vi "Apply Bounds.vi"(8 "error in":errorcluster, 10 "Bounds":refnum<class "Vec3d.lvclass">, 11 "Vec3d in":refnum<class "Vec3d.lvclass">) -> (0 "error out":errorcluster, 3 "Vec3d out":refnum<class "Vec3d.lvclass">)   [LabVIEW 2017, in "Vec3d.lvclass"]
doc: "Shrinks the vector if necessary so the magnitude of all components are less than the corresponding components of the Bounds Vec3d. All components are scaled equally so the direction of the vector will not change"
uses:
  Vec3d.lvclass
  Vec3d.lvclass/Vec3d.ctl
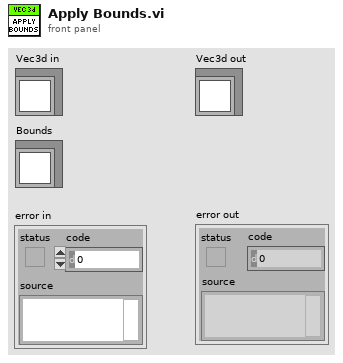
[diagram p1: front panel]
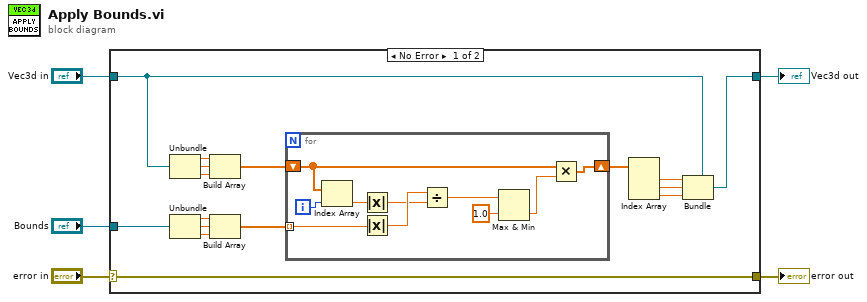
[diagram p0: block diagram]
diagram:
  n1 = case shown="No Error" "error in" {
    selector: "error in" -> [w21 w33]
    tunnel: [w21 w33] -> w4
    tunnel: [w6 w32] -> w2
    tunnel: "Vec3d in" -> [w7 w32]
    tunnel: "Bounds" -> [w20 _]
    frame No Error {
      n2 = Unbundle(w7) -> (w12:dbl, w14:dbl, w15:dbl)
      n3 = Unbundle(w20) -> (w19:dbl, w18:dbl, w17:dbl)
      n4 = Build Array(w12, w14, w15) -> (w13:dbl[])
      n5 = Build Array(w19, w18, w17) -> (w16:dbl[])
      n6 = for {
        tunnel: w16 -> [w30] mode=indexing
        shift-right: [w22] -> w11
        shift-left: w13 -> [w24]
        i -> [w31]
        n7 = Index Array(array=w24, index=w31) -> (element=w29:dbl)
        n8 = Absolute Value(x=w29) -> (abs(x)=w27:dbl)
        n9 = Absolute Value(x=w30) -> (abs(x)=w28:dbl)
        n10 = Divide(x=w28, y=w27) -> (x/y=w26:dbl)
        n11 = Max & Min(x=w26, y=1.0) -> (min(x,y)=w23:dbl)  [unwired: 1 out]
        n12 = Multiply(x=w24, y=w23) -> (x*y=w22:dbl[])
      }
      n13 = Index Array(array=w11) -> (element #1=w10:dbl, element #2=w9:dbl, element #3=w8:dbl)  [unwired: 3 in]
      n14 = Bundle(cluster=w7, w10, w9, w8) -> (w6:refnum<class "Vec3d.lvclass">)
    }
    frame Error {
    }
  }
  "error out" <- w4
  "Vec3d out" <- w2
